vi "pb-read_status.vi"(8 "error in (no error)":errorcluster, 11 "path in":path=path "C:/SpinCore/SpinAPI/dll/spinapi64.dll") -> (0 "error out":errorcluster, 2 "status":T1, 3 "path out":path)   [LabVIEW 2018]
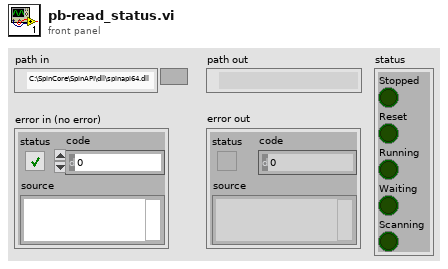
[diagram p1: front panel]
types:
  T1 = cluster{"Stopped":bool, "Reset":bool, "Running":bool, "Waiting":bool, "Scanning":bool}
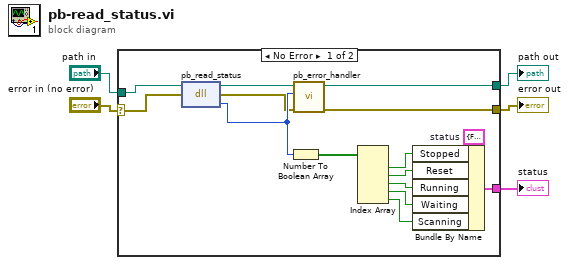
[diagram p0: block diagram]
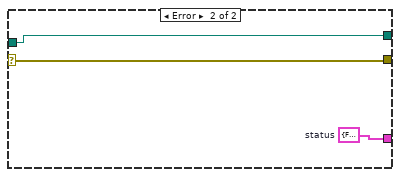
[diagram p2: hidden frame]
diagram:
  n1 = case shown="No Error" "error in (no error)" {
    selector: "error in (no error)" -> [w10 w22]
    tunnel: "path in" -> [w7 w23]
    tunnel: [w20 w23] -> w2
    tunnel: [w19 w22] -> w3
    tunnel: [w12 w21] -> w1
    frame No Error {
      w18 = T1 {"Stopped"=FALSE, "Reset"=FALSE, "Running"=FALSE, "Waiting"=FALSE, "Scanning"=FALSE}  # status
      n2 = dll-call lib="C:/SpinCore/SpinAPI/lib/spinapi64.dll" fn="pb_read_status"(path in=w7, error in=w10) -> (path out=w8:path, error out=w9:errorcluster, "return type"=w11:i32)  [unwired: 1 in]
      n3 = Number To Boolean Array(number=w11) -> (Boolean array=w6:bool[])
      n4 = call "pb_error_handler.vi"("error in (no error)"=w9, "return code"=w11, "path in"=w8) -> ("error out"=w19:errorcluster, "path out"=w20:path)  [unwired: 7 in]
      n5 = Index Array(array=w6) -> (element #1=w17:bool, element #2=w16:bool, element #3=w15:bool, element #4=w14:bool, element #5=w13:bool)  [unwired: 5 in]
      n6 = Bundle By Name(cluster=w18, "Stopped"=w17, "Reset"=w16, "Running"=w15, "Waiting"=w14, "Scanning"=w13) -> (w12:T1)
    }
    frame Error {
      w21 = T1 {"Stopped"=FALSE, "Reset"=FALSE, "Running"=FALSE, "Waiting"=FALSE, "Scanning"=FALSE}  # status
    }
  }
  "path out" <- w2
  "error out" <- w3
  "status" <- w1
